vi "GetEvents.vi"(8 "error in (no error)":errorcluster, 11 "ICameraTesting in":refnum<class "ICameraTesting.lvclass">) -> (0 "error out":errorcluster, 2 "CameraTestingEvnt":T1, 3 "ICameraTesting out":refnum<class "ICameraTesting.lvclass">)   [LabVIEW 2020, in "ICameraTesting.lvlib" / "ICameraTesting.lvclass"]
uses:
  ICameraTesting.lvclass
  Camera/ICamera/ICamera/TypeDef/SnapInfo.ctl
  Camera/ICamera/ICamera/ICamera.lvclass
  TypeDef/FrameRateValReceived.ctl
  TypeDef/ImgTypeValReceived.ctl
  TypeDef/ResolutionValReceived.ctl
  TypeDef/Events.ctl
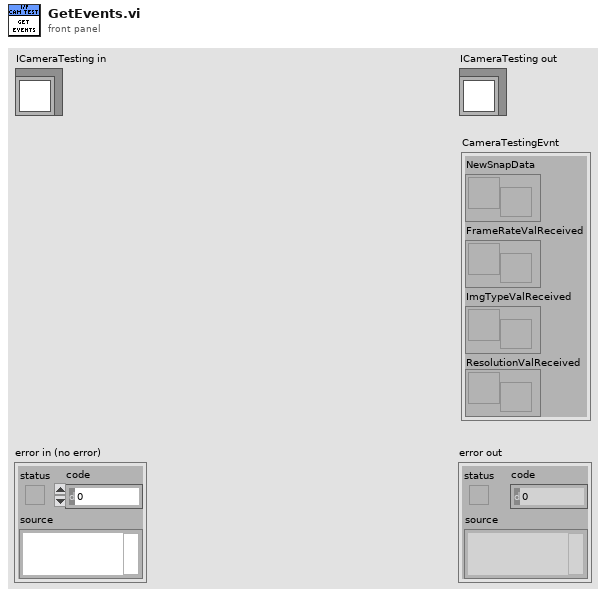
[diagram p1: front panel]
types:
  T1 = typedef "ICameraTesting.lvlib/ICameraTesting.lvclass/Events.ctl" = cluster{"NewSnapData":refnum<user-event>, "FrameRateValReceived":T2, "ImgTypeValReceived":T3, "ResolutionValReceived":T4}
  T2 = typedef "ICameraTesting.lvlib/ICameraTesting.lvclass/FrameRateValReceived.ctl" = refnum<user-event>
  T3 = typedef "ICameraTesting.lvlib/ICameraTesting.lvclass/ImgTypeValReceived.ctl" = refnum<user-event>
  T4 = typedef "ICameraTesting.lvlib/ICameraTesting.lvclass/ResolutionValReceived.ctl" = refnum<user-event>
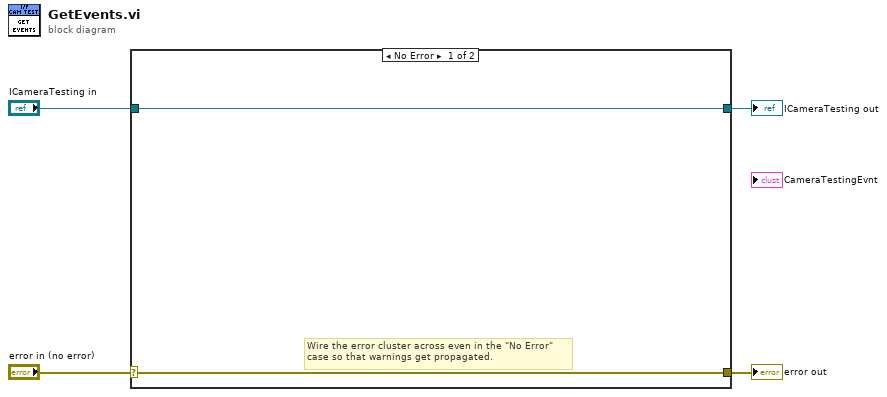
[diagram p0: block diagram]
diagram:
  n1 = case shown="No Error" "error in (no error)" {
    selector: "error in (no error)" -> [w5 w8]
    tunnel: [w5 w8] -> w3
    tunnel: [w6 w7] -> w1
    tunnel: "ICameraTesting in" -> [w6 w7]
    frame No Error {
      # "Wire the error cluster across even in the \"No Error\"\ncase so that warnings get propagated."
    }
    frame Error {
    }
  }
  "error out" <- w3
  "ICameraTesting out" <- w1
